vi "send_array_to_python.vi"() -> ()   [LabVIEW 2014]
panel:
  out "python input":string
  out "standard error":string
  out "error out":errorcluster
  out "python output":string
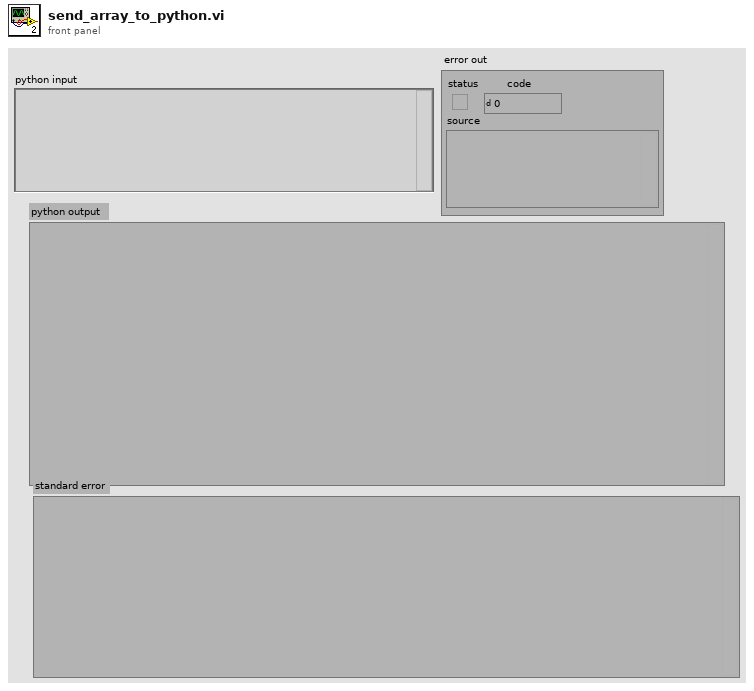
[diagram p1: front panel]
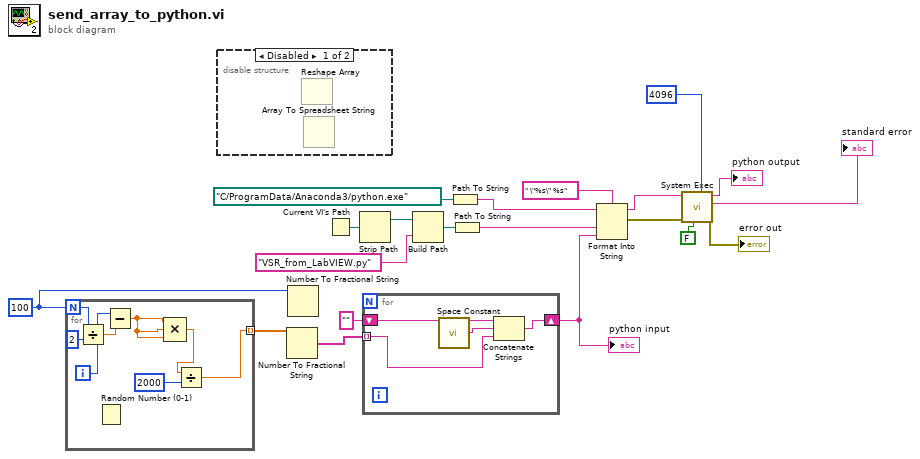
[diagram p0: block diagram]
diagram:
  w8 = 100
  n1 = for {
    N: w8 -> [w24]
    tunnel: [w27] -> w2 mode=indexing
    i -> [w26]
    n2 = Divide(x=w24, y=2) -> (x/y=w25:dbl)
    n3 = Random Number (0-1)() -> ()  [unwired: 1 out]
    n4 = Subtract(x=w26, y=w25) -> (x-y=w21:dbl)
    n5 = Compound Arithmetic op=MULTIPLY(w21, w21, w21) -> (w22:dbl)
    n6 = Divide(x=w22, y=2000) -> (x/y=w27:dbl)
  }
  n7 = disable-structure shown="Disabled" {
    frame Disabled {
      n8 = Reshape Array() -> ()  [unwired: 2 in, 1 out]
      n9 = Array To Spreadsheet String() -> ()  [unwired: 3 in, 1 out]
    }
    frame Enabled {
    }
  }
  n10 = Number To Fractional String(number=w2) -> (F-format string=w11:string[])  [unwired: 3 in]
  n11 = Number To Fractional String(number=w8) -> ()  [unwired: 3 in, 1 out]
  n12 = Current VI's Path() -> (path=w17:path)
  n13 = Strip Path(path=w17) -> (stripped path=w15:path)  [unwired: 1 out]
  n14 = for {
    tunnel: w11 -> [w30] mode=indexing
    shift-right: [w31] -> w4
    shift-left: "" -> [w29]
    n15 = call <vilib>:"Space Constant.vi"() -> ("String"=w32:string)
    n16 = Concatenate Strings(w29, w32, w30) -> (w31:string)
  }
  "python input" <- w4
  n17 = Build Path(base path=w15, name or relative path="VSR_from_LabVIEW.py" ("Path to Function")) -> (appended path=w18:path)
  n18 = Path To String(path=path "C:/ProgramData/Anaconda3/python.exe" ("Path to Python.exe")) -> (string=w12:string)
  n19 = Path To String(path=w18) -> (string=w7:string)
  n20 = Format Into String(format string=" \"%s\" %s", initial string=w12, w7, w4) -> (resulting string=w10:string, error out=w9:errorcluster)  [unwired: 1 in]
  n21 = call <vilib>:"System Exec.vi"("expected output size  (4096)"=u32 4096, "run minimized? (F)"=FALSE, "error in (no error)"=w9, "command line"=w10) -> ("error out"=→"error out":errorcluster, "standard error"=→"standard error":string, "standard output"=→"python output":string)  [unwired: 4 in, 1 out]
